vi "ScriptSetIcon.vi"(6 "numeric representation":T1=enum."Word", 8 "error in (no error)":errorcluster, 9 "digital(F)/numeric(T)":bool, 10 "indicator (F)/control (T)":bool, 11 "VI reference":refnum<vi>) -> (0 "error out":errorcluster, 3 "VI reference out":refnum<vi>)   [LabVIEW 2014]
uses:
  <vilib>/numeric/LVNumericRepresentation.ctl
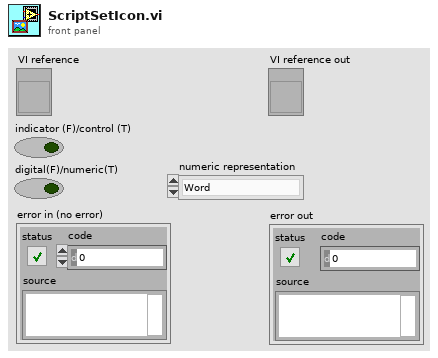
[diagram p1: front panel]
types:
  T1 = typedef "LVNumericRepresentation.ctl" = enum32{"Extended Precision", "Double Precision", "Single Precision", "Long", "Word", "Byte", "Unsigned Long", "Unsigned Word", "Unsigned Byte", "Complex Extended", "Complex Double", "Complex Single", "Quad", "Unsigned Quad", "Fixed-Point"}
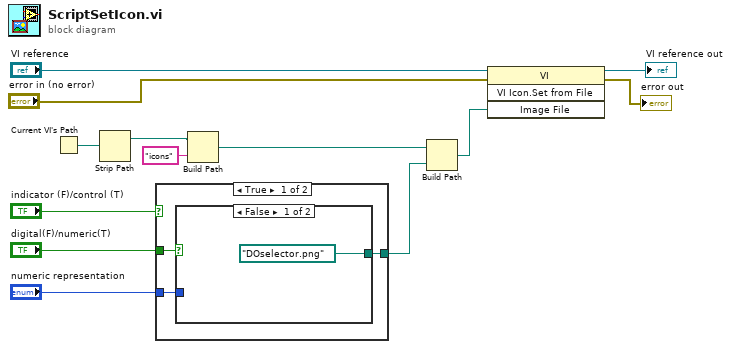
[diagram p0: block diagram]
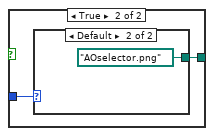
[diagram p2: hidden frame]
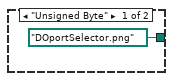
[diagram p3: hidden frame]
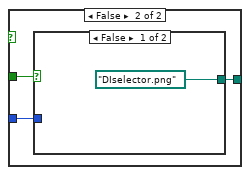
[diagram p4: hidden frame]
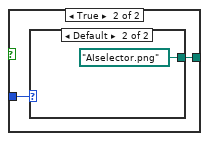
[diagram p5: hidden frame]
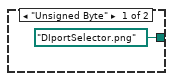
[diagram p6: hidden frame]
diagram:
  n1 = Current VI's Path() -> (path=w9:path)
  n2 = Strip Path(path=w9) -> (stripped path=w8:path)  [unwired: 1 out]
  n3 = case shown="True" "indicator (F)/control (T)" {
    tunnel: "digital(F)/numeric(T)" -> [w16 w24]
    tunnel: "numeric representation" -> [w15 w23]
    tunnel: [w14 w22] -> w1
    frame True {
      n4 = case shown="False" w16 {
        tunnel: w15 -> [_ w18]
        tunnel: [path "DOselector.png" ("Path") w19] -> w14
        frame False {
        }
        frame True {
          n5 = case shown="Default" w18 {
            tunnel: [path "DOportSelector.png" ("Path") path "AOselector.png" ("Path")] -> w19
            frame "Unsigned Byte" {
            }
            frame Default {
            }
          }
        }
      }
    }
    frame False {
      n6 = case shown="False" w24 {
        tunnel: w23 -> [_ w27]
        tunnel: [path "DIselector.png" ("Path") w26] -> w22
        frame False {
        }
        frame True {
          n7 = case shown="Default" w27 {
            tunnel: [path "DIportSelector.png" ("Path") path "AIselector.png" ("Path")] -> w26
            frame "Unsigned Byte" {
            }
            frame Default {
            }
          }
        }
      }
    }
  }
  n8 = Build Path(base path=w8, name or relative path="icons") -> (appended path=w2:path)
  n9 = Build Path(base path=w2, name or relative path=w1) -> (appended path=w3:path)
  n10 = invoke class="VI" method="VI Icon.Set from File"(reference="VI reference", error in="error in (no error)", "Image File"=w3) -> (reference out=→"VI reference out":refnum<vi>, error out=→"error out":errorcluster)  [unwired: 1 in, 2 out]
